vi "Streaming Example.vi"() -> ()   [LabVIEW 2024]
uses:
  Sift API/Sift Client.lvclass
  Generate Sift Protos/SiftProxy_client/RPC Messages/sift_proxy_v1_ChannelDataType.ctl
  Generate Sift Protos/SiftProxy_client/SiftProxy_client.lvlib
  Sift Client.lvlib
panel:
  out "Flush Error":errorcluster
  in  "Test Channel 2":dbl(slide) scale=0.0..10.0
  in  "Stop":bool
  in  "Test Channel 1":dbl(slide) scale=0.0..10.0
  in  "Test Channel 3":bool
  out "runId":string
  in  "Run Name":string
  out "error out":errorcluster
  in  "Organization ID":string
  in  "API Key":string
  in  "API URL":string
  # "Sift Streaming Example"
  # "This example streams data live from LabVIEW.\n\nFill in the information below then open the corresponding Run in Sift\nto see data streaming in Live.\n\nNote: Remembver to hit the \"Live\" button after opening the run."
  # "Adjust these values while streaming"
  # "Hit this to stop the example."
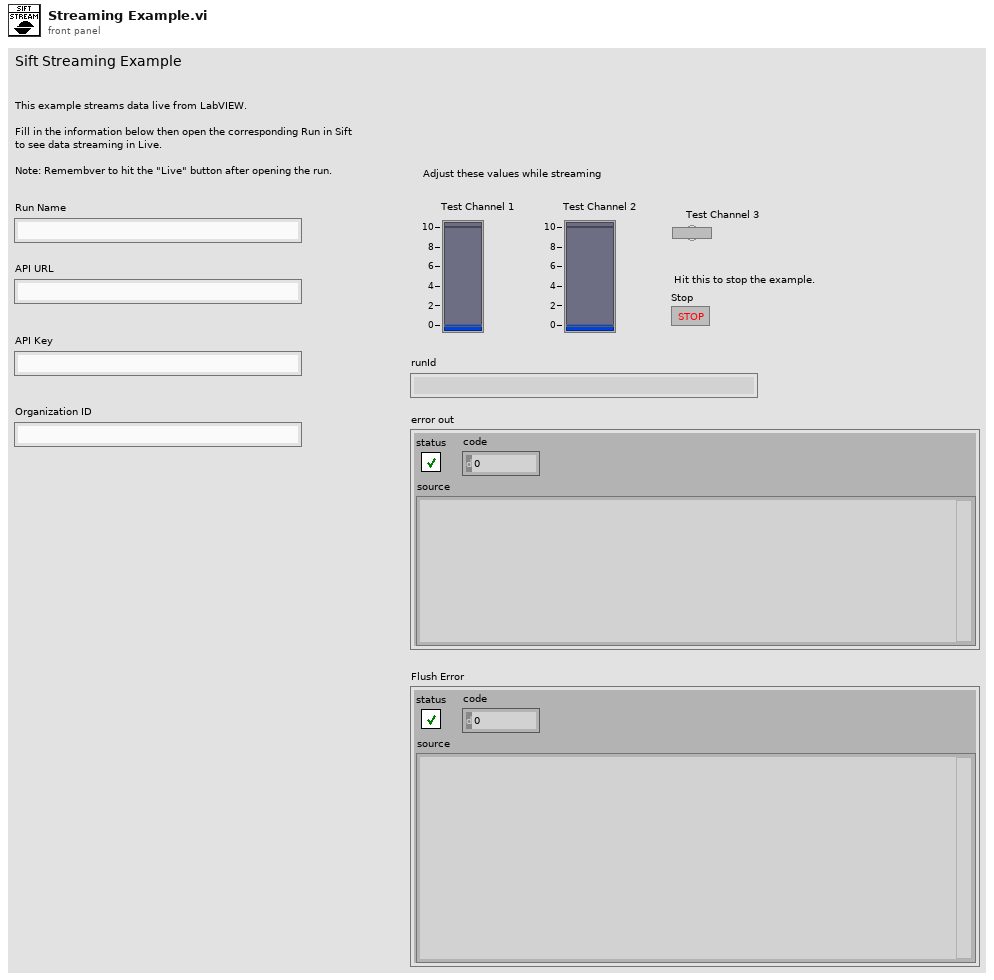
[diagram p1: front panel]
types:
  T1 = typedef "SiftProxy_client.lvlib/sift_proxy_v1_ChannelDataType.ctl" = enum32{"CHANNEL_DATA_TYPE_UNSPECIFIED", "CHANNEL_DATA_TYPE_DOUBLE", "CHANNEL_DATA_TYPE_STRING", "CHANNEL_DATA_TYPE_ENUM", "CHANNEL_DATA_TYPE_BIT_FIELD", "CHANNEL_DATA_TYPE_BOOL", "CHANNEL_DATA_TYPE_FLOAT", "CHANNEL_DATA_TYPE_INT_32", "CHANNEL_DATA_TYPE_UINT_32", "CHANNEL_DATA_TYPE_INT_64", "CHANNEL_DATA_TYPE_UINT_64"}
  T2 = typedef "SiftProxy_client.lvlib/google_protobuf_Timestamp.ctl" = cluster{"seconds":i64, "nanos":i32}
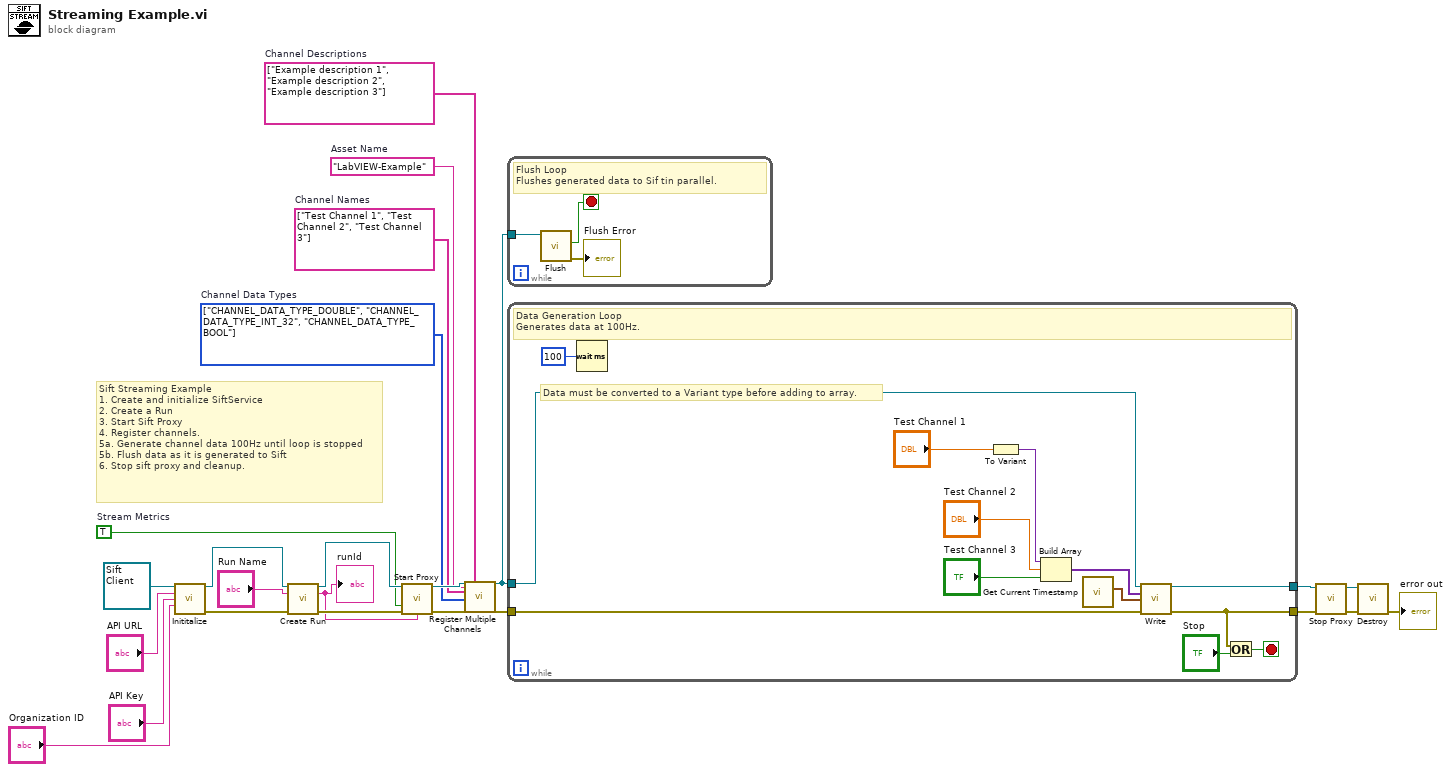
[diagram p0: block diagram]
diagram:
  w6 = "LabVIEW-Example"  # Asset Name
  w8 = T1[] [enum."CHANNEL_DATA_TYPE_DOUBLE", enum."CHANNEL_DATA_TYPE_INT_32", enum."CHANNEL_DATA_TYPE_BOOL"] items=["CHANNEL_DATA_TYPE_UNSPECIFIED", "CHANNEL_DATA_TYPE_DOUBLE", "CHANNEL_DATA_TYPE_STRING", "CHANNEL_DATA_TYPE_ENUM", "CHANNEL_DATA_TYPE_BIT_FIELD", "CHANNEL_DATA_TYPE_BOOL", "CHANNEL_DATA_TYPE_FLOAT", "CHANNEL_DATA_TYPE_INT_32", "CHANNEL_DATA_TYPE_UINT_32", "CHANNEL_DATA_TYPE_INT_64", "CHANNEL_DATA_TYPE_UINT_64"]  # Channel Data Types
  w7 = string[] ["Example description 1", "Example description 2", "Example description 3"]  # Channel Descriptions
  w9 = string[] ["Test Channel 1", "Test Channel 2", "Test Channel 3"]  # Channel Names
  w15 = TRUE  # Stream Metrics
  # "Sift Streaming Example\n1. Create and initialize SiftService\n2. Create a Run\n3. Start Sift Proxy\n4. Register channels.\n5a. Generate channel data 100Hz until loop is stopped\n5b. Flush data as it is generated to Sift\n6. Stop sift proxy and cleanup."
  n1 = call-dynamic "Inititalize.vi"("Sift Client in"=refnum<class "Sift Client.lvclass"> refnum ("Sift Client.lvlib:Sift Client.lvclass"), "API URL"="API URL", "API Key"="API Key", "Organization ID"="Organization ID") -> ("Sift Client out"=w20:refnum<class "Sift Client.lvclass">, "error out"=w18:errorcluster)  [unwired: 10 in]
  n2 = call-dynamic "Create Run.vi"("Sift Client in"=w20, "name"="Run Name", "error in (no error)"=w18) -> ("Sift Client out"=w19:refnum<class "Sift Client.lvclass">, "runId"=w2:string, "error out"=w16:errorcluster)  [unwired: 10 in]
  "runId" <- w2
  n3 = call-dynamic "Start Proxy.vi"("Sift Client in"=w19, "Stream Metrics"=w15, "error in (no error)"=w16, "Run ID"=w2) -> ("Sift Client out"=w10:refnum<class "Sift Client.lvclass">, "error out"=w11:errorcluster)  [unwired: 10 in]
  n4 = call "Register Multiple Channels.vi"("Sift Client in"=w10, "Asset Name"=w6, "Names"=w9, "Data Types"=w8, "error in (no error)"=w11, "Descriptions"=w7) -> ("Sift Client out"=w1:refnum<class "Sift Client.lvclass">, "error out"=w5:errorcluster)  [unwired: 20 in]
  n5 = while {
    tunnel: w1 -> [w27]
    stop <- w26 stop-if-true
    # "Flush Loop\nFlushes generated data to Sif tin parallel."
    n6 = call-dynamic "Flush.vi"("Sift Client in"=w27) -> ("error out"=→"Flush Error":errorcluster, "Done"=w26:bool)  [unwired: 8 in, 1 out]
  }
  n7 = while {
    tunnel: w1 -> [w40]
    tunnel: w5 -> [w39]
    tunnel: [w32] -> w4
    tunnel: [w34] -> w3
    stop <- w31 stop-if-true
    # "Data must be converted to a Variant type before adding to array."
    # "Data Generation Loop\nGenerates data at 100Hz."
    n8 = Wait (ms)(milliseconds to wait=u32 100) -> ()  [unwired: 1 out]
    n9 = To Variant(anything="Test Channel 1") -> (Variant=w37:variant)
    n10 = Build Array(w37, "Test Channel 2", "Test Channel 3") -> (w36:variant[])
    n11 = call "Get Current Timestamp.vi"() -> ("Timestamp"=w35:T2)  [unwired: 11 in]
    n12 = call-dynamic "Write.vi"("Sift Client in"=w40, "Values"=w36, "Timestamp"=w35, "error in (no error)"=w39) -> ("Sift Client out"=w32:refnum<class "Sift Client.lvclass">, "error out"=w34:errorcluster)  [unwired: 10 in]
    n13 = Or(x=w34, y="Stop") -> (x .or. y?=w31:bool)
  }
  n14 = call-dynamic "Stop Proxy.vi"("error in (no error)"=w3, "Sift Client in"=w4) -> ("error out"=w14:errorcluster, "Sift Client out"=w13:refnum<class "Sift Client.lvclass">)  [unwired: 8 in]
  n15 = call-dynamic "Destroy.vi"("error in (no error)"=w14, "Sift Client in"=w13) -> ("error out"=→"error out":errorcluster)  [unwired: 8 in, 1 out]
